vi "calibrationElectrometer_logEvent_settingsAppliedSerConf.vi"(8 "error in (no error)":errorcluster, 11 "logevent_settingsAppliedSerConf_Ctl":T1={"visaResource"="", "baudRate"=0, "parity"=0, "dataBits"=0, "stopBits"=0, "flowControl"=0, "termChar"=0, "electId"="                                                                                                                                                                                                                                                                ", "priority"=0}) -> (0 "error out":errorcluster, 2 "function return":i32, 3 "logevent_settingsAppliedSerConf_Ctl out":T1={"visaResource"="", "baudRate"=0, "parity"=0, "dataBits"=0, "stopBits"=0, "flowControl"=0, "termChar"=0, "electId"="                                                                                                                                                                                                                                                                ", "priority"=0})   [LabVIEW 2016, in "SALLV_calibrationElectrometer.lvlib"]
doc: "int calibrationElectrometer_shm_logEvent_settingsAppliedSerConfLV(calibrationElectrometer_logevent_settingsAppliedSerConfLV *logevent_settingsAppliedSerConf_Ctl );"
uses:
  SALLV_calibrationElectrometer.lvlib
  DataTypes/logevent_settingsAppliedSerConf.ctl
  SALLV_calibrationElectrometer.so
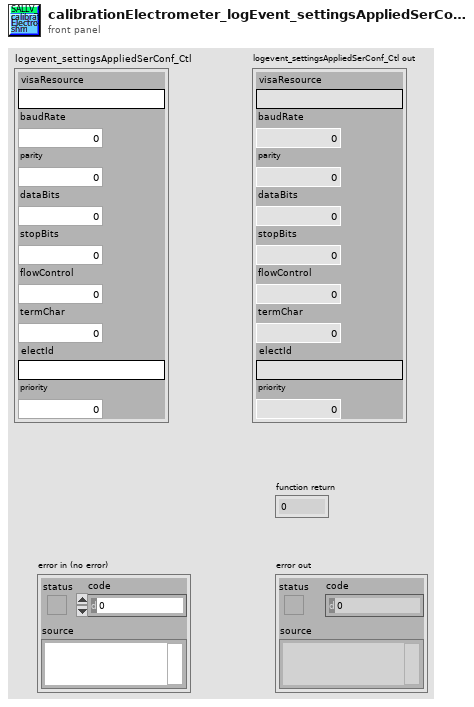
[diagram p1: front panel]
types:
  T1 = typedef "SALLV_calibrationElectrometer.lvlib/logevent_settingsAppliedSerConf.ctl" = cluster{"visaResource":string, "baudRate":i32, "parity":i32, "dataBits":i32, "stopBits":i32, "flowControl":i32, "termChar":i32, "electId":string, "priority":i32}
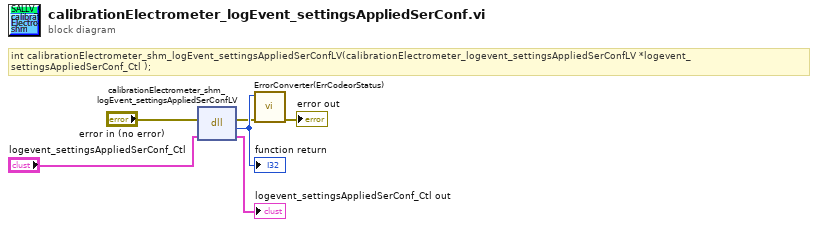
[diagram p0: block diagram]
diagram:
  # "int calibrationElectrometer_shm_logEvent_settingsAppliedSerConfLV(calibrationElectrometer_logevent_settingsAppliedSerConfLV *logevent_settingsAppliedSerConf_Ctl );"
  n1 = dll-call lib="home/andres/Desktop/SAL_calibrationElectrometer/SALLV_calibrationElectrometer.*" fn="calibrationElectrometer_shm_logEvent_settingsAppliedSerConfLV"(error in="error in (no error)", "logevent_settingsAppliedSerConf_Ctl"="logevent_settingsAppliedSerConf_Ctl") -> (error out=w2:errorcluster, w6:i32, "logevent_settingsAppliedSerConf_Ctl"=→"logevent_settingsAppliedSerConf_Ctl out":T1)  [unwired: 2 in, 1 out]
  "function return" <- w6
  n2 = call "ErrorConverter(ErrCodeorStatus).vi"("error in (no error)"=w2, "error code"=w6) -> ("error out"=→"error out":errorcluster)  [unwired: 9 in]
